vi "manual_comparison.vi"(8 "error in (no error)":errorcluster, 11 "data":variant) -> (0 "error out":errorcluster)   [LabVIEW 2015, in "example_01.lvlib"]
uses:
  example_01.lvlib
  _controls/steps_actions_data.ctl
  _controls/steps_actions.ctl
  <userlib>/antonio-alexander/lv-recipe-machine/lv-recipe-machine.lvlib
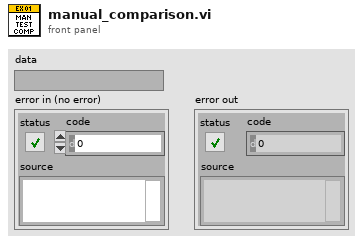
[diagram p1: front panel]
types:
  T1 = typedef "example_01.lvlib/steps_actions.ctl" = enum16{"<steps_actions>", "manual_random", "manual_comparison", "manual_wait", "auto_random", "auto_wait", "criteria_initialize", "criteria_count", "criteria_comparison", "transition_simple", "transition_count", "transition_comparison", "launch_wait", "<null>"}
  T2 = typedef "example_01.lvlib/steps_actions_data.ctl" = cluster{"step_action":T1, "data":variant}
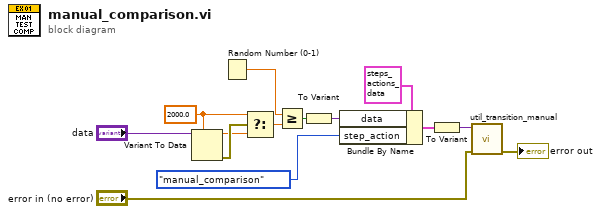
[diagram p0: block diagram]
diagram:
  w9 = 2000.0
  n1 = Variant To Data(type=w9, Variant="data") -> (data=w8:dbl, error out=w10:errorcluster)  [unwired: 1 in]
  n2 = Random Number (0-1)() -> (number: 0 to 1=w1:dbl)
  n3 = Select(t=w9, s=w10, f=w8) -> (s? t:f=w2:dbl)
  n4 = Greater Or Equal?(x=w1, y=w2) -> (x >= y?=w7:bool)
  n5 = To Variant(anything=w7) -> (Variant=w12:variant)
  n6 = Bundle By Name(cluster=T2 {"step_action"=enum."<steps_actions>", "data"=variant}, "data"=w12, "step_action"=steps_actions."manual_comparison" ("manual_action")) -> (w6:T2)
  n7 = To Variant(anything=w6) -> (Variant=w5:variant)
  n8 = call <userlib>:"util_transition_manual.vi"("error in (no error)"="error in (no error)", "data"=w5) -> ("error out"=→"error out":errorcluster)  [unwired: 9 in]
